vi "Flush Data to Log File.vi"(8 "error in (no error)":errorcluster, 11 "Logging Configuration":T1={"Log File Base Path"=path "", "TDMS File Reference"=refnum, "Reset"=FALSE, "Wait"=0.0, "Start Time"=0.0, "Update Rate"=1, "Channel Names"=[], "System Preset"=variant} {"Update Rate" min=1 max=10 step=1}) -> (0 "error out":errorcluster, 3 "file path out":path)   [LabVIEW 2020, in "SAVE.lvlib"]
doc: "Flush the data queue of any pending data and write it to the log file. Close the TDMS file reference."
uses:
  SAVE.lvlib
  Save Configuration.ctl
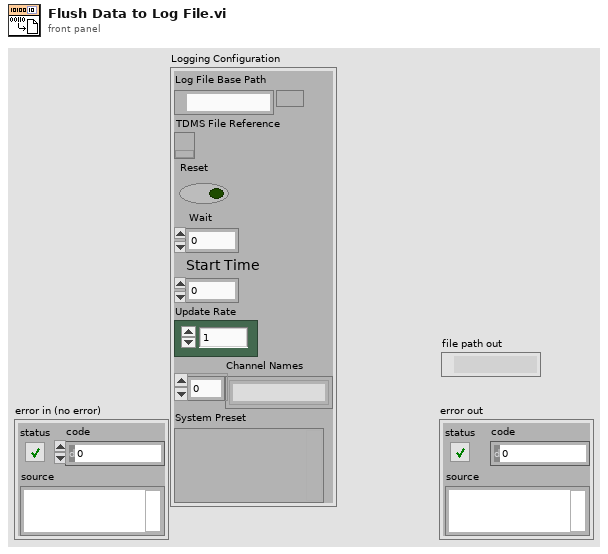
[diagram p1: front panel]
types:
  T1 = typedef "SAVE.lvlib/Save Configuration.ctl" = cluster{"Log File Base Path":path, "TDMS File Reference":refnum<k34>, "Reset":bool, "Wait":dbl, "Start Time":dbl, "Update Rate":u16, "Channel Names":string[], "System Preset":variant}
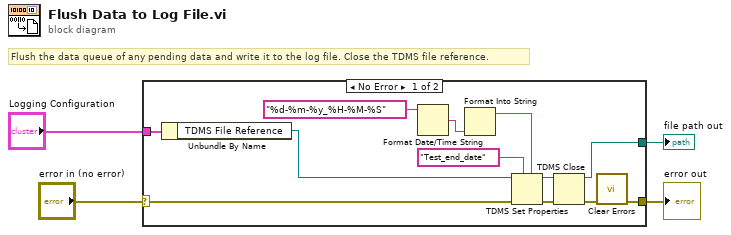
[diagram p0: block diagram]
diagram:
  # "Flush the data queue of any pending data and write it to the log file. Close the TDMS file reference."
  n1 = case shown="No Error" "error in (no error)" {
    selector: "error in (no error)" -> [w6 w17]
    tunnel: "Logging Configuration" -> [w16 _]
    tunnel: [w14 w17] -> w3
    tunnel: [w13 _] -> w1
    frame No Error {
      n2 = Unbundle By Name(w16) -> ("TDMS File Reference"=w10:refnum<k34>)
      n3 = Format Date/Time String(time format string (%c)="%d-%m-%y_%H-%M-%S") -> (date/time string=w11:string)  [unwired: 2 in]
      n4 = Format Into String(w11) -> (resulting string=w7:string)  [unwired: 3 in, 1 out]
      n5 = TDMS Set Properties(5:w7, 7:"Test_end_date" ("time format string (%c)"), 8:w6, 11:w10) -> (0:w5:errorcluster, 3:w9:refnum<k34>)  [unwired: 2 in, 2 out]
      n6 = TDMS Close(8:w5, 11:w9) -> (0:w15:errorcluster, 3:w13:path)
      n7 = call <vilib>:"Clear Errors.vi"("error in (no error)"=w15) -> ("error out"=w14:errorcluster)  [unwired: 5 in, 1 out]
    }
    frame Error {
    }
  }
  "error out" <- w3
  "file path out" <- w1
